vi "Create Host Stream Refs.vi"(8 "error in (no error)":errorcluster, 10 "Addon":string, 11 "Target IP Address":string) -> (0 "error out":errorcluster, 3 "Refs":T1)   [LabVIEW 2019, in "CAN Streaming Support Workspace Shared.lvlib"]
uses:
  CAN Streaming Support Workspace Shared.lvlib
  Types/Host Stream API Refs.ctl
  <vilib>/xnet/xnet.llb/XNET Frame CAN.ctl
  <vilib>/xnet/xnet.llb/XNET Frame Type CAN.ctl
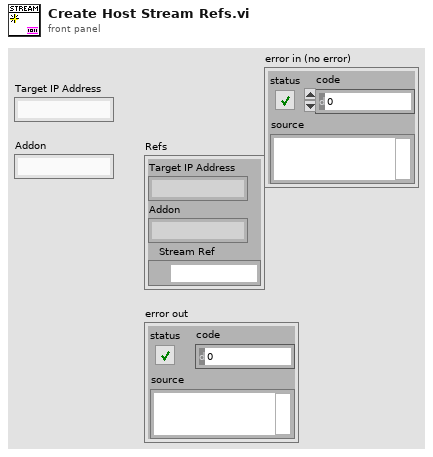
[diagram p1: front panel]
types:
  T1 = typedef "CAN Streaming Support Workspace Shared.lvlib/Host Stream API Refs.ctl" = cluster{"Target IP Address":string, "Addon":string, "Stream Ref":refnum<k21>}
  T2 = typedef "XNET Frame CAN.ctl" = cluster{"timestamp":timestamp, "payload":u8[], "identifier":u32, "type":T3, "extended?":bool, "echo?":bool}
  T3 = typedef "XNET Frame Type CAN.ctl" = u8
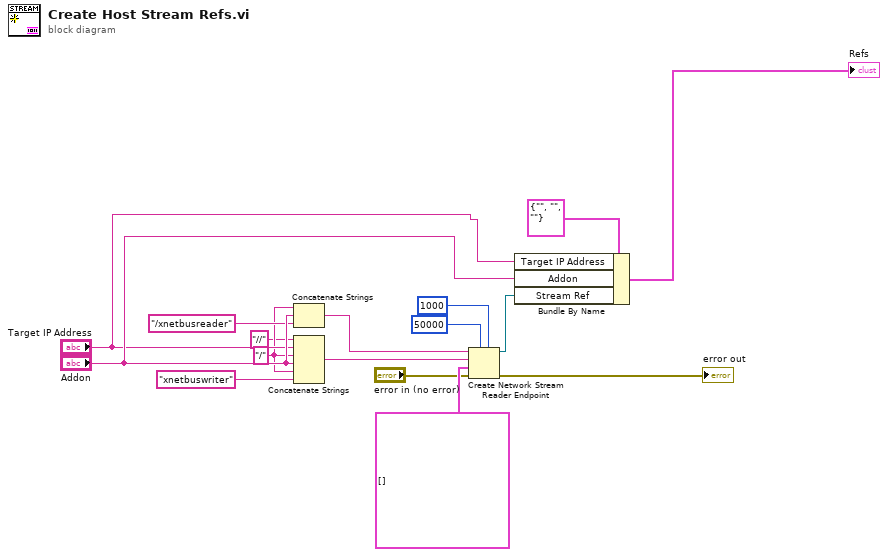
[diagram p0: block diagram]
diagram:
  w8 = "/" ("string")
  n1 = Concatenate Strings(w8, "Addon", "/xnetbusreader" ("writer name")) -> (w10:string)
  n2 = Concatenate Strings("//" ("reader url"), "Target IP Address", w8, "Addon", w8, "xnetbuswriter" ("reader url")) -> (w7:string)
  n3 = Create Network Stream Reader Endpoint(5:1000 ("timeout in ms (-1)"), 7:50000 ("reader buffer size"), 8:"error in (no error)", 9:T2[] [] ("CAN Frame Input"), 10:w7, 11:w10) -> (0:→"error out":errorcluster, 3:w14:refnum<k21>)  [unwired: 1 in]
  n4 = Bundle By Name(cluster=T1 {"Target IP Address"="", "Addon"="", "Stream Ref"=""}, "Target IP Address"="Target IP Address", "Addon"="Addon", "Stream Ref"=w14) -> (→"Refs":T1)
